vi "Stop Core.vi"(10 "final error code":i32, 11 "UDP_transmitter in":refnum<class "UDP_transmitter.lvclass">) -> (3 "UDP_transmitter out":refnum<class "UDP_transmitter.lvclass">)   [LabVIEW 2025, in "UDP_transmitter.lvlib" / "UDP_transmitter.lvclass"]
doc: "(<B>Filename</B>: Actor Framework.lvlib:Actor.lvclass:Stop Core.vi)\n\nDefines what the actor does before it stops. Use the <B>final error code</B> input to determine whether the actor shut down in response to an error.\n\nBy default, this method passes the Stop message along to all auto-stop nested actors. A descendant class may override this method to define additional behavior, such as shutting down any processes the actor initiated in its override of the Actor Core method."
uses:
  UDP_transmitter.lvclass
  UDP_transmitter.lvclass/UDP_transmitter.ctl
  <vilib>/ActorFramework/Actor/Actor.lvclass
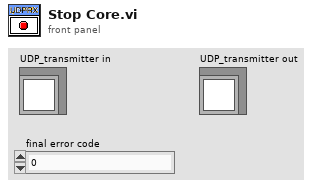
[diagram p1: front panel]
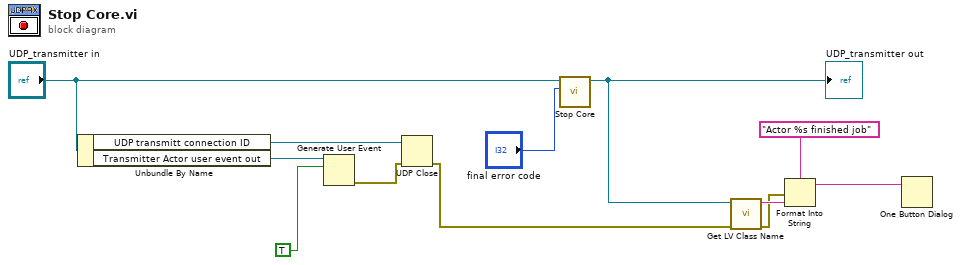
[diagram p0: block diagram]
diagram:
  n1 = Unbundle By Name("UDP_transmitter in") -> ("UDP transmitt connection ID"=w10:refnum<k16>, "Transmitter Actor user event out"=w5:refnum<user-event>)
  n2 = Generate User Event(user event=w5, event data cluster=TRUE ("event data")) -> (error out=w3:errorcluster)  [unwired: 2 in, 1 out]
  n3 = UDP Close(connection ID=w10, 8:w3) -> (error out=w2:errorcluster)  [unwired: 1 out]
  n4 = call-parent "Stop Core.vi"("final error code"="final error code", "Actor in"="UDP_transmitter in") -> ("Actor out"=w6:refnum<class "UDP_transmitter.lvclass">)  [unwired: 9 in]
  "UDP_transmitter out" <- w6
  n5 = call <vilib>:"Get LV Class Name.vi"("error in (no error)"=w2, "object"=w6) -> ("error out"=w1:errorcluster, "class name"=w9:string)  [unwired: 8 in]
  n6 = Format Into String(format string="Actor %s finished job", error in=w1, w9) -> (resulting string=w7:string)  [unwired: 1 in, 1 out]
  n7 = One Button Dialog(message=w7) -> ()  [unwired: 1 in, 1 out]
